vi "ADIS16470 Process AutoSPI DMA.vi"(8 "error in (no error)":T1, 9 "Bytes per Sample":numeric, 10 "Samples to Read":numeric) -> (0 "error out":T1, 1 "Timestamps":array[numeric], 2 "Data":array[numeric])   [LabVIEW 2019]
uses:
  <vilib>/Utility/error.llb/Error Cluster From Error Code.vi
  <vilib>/rvi/errors/niLvFpgaAdjustHostInterfaceError.vi
  <vilib>/rvi/interface/nirviMethod/nirviMethod.xnode
  <vilib>/Rock Robotics/SystemInterfaces/System/FPGA_SystemFRC FPGA Ref.ctl
  <vilib>/FPGAPlugInAG/Dynamic/niLvFpga_ReadFifo_Dynamic.vi
  <vilib>/rvi/errors/niLvFpgaMergeErrorWithErrorCode.vi
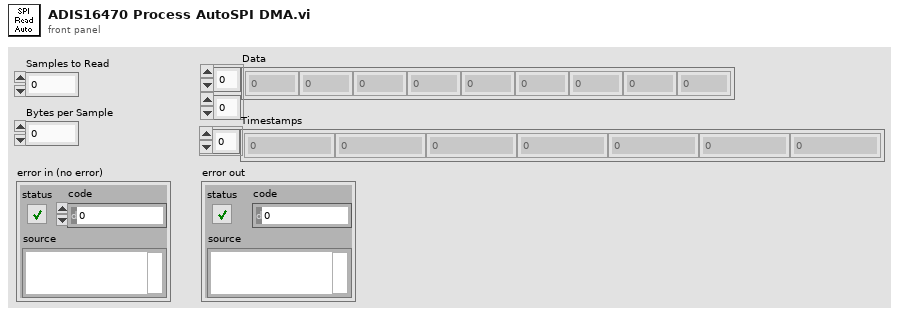
[diagram p1: front panel]
types:
  T1 = cluster{"source":string, "code":numeric, "status":boolean}
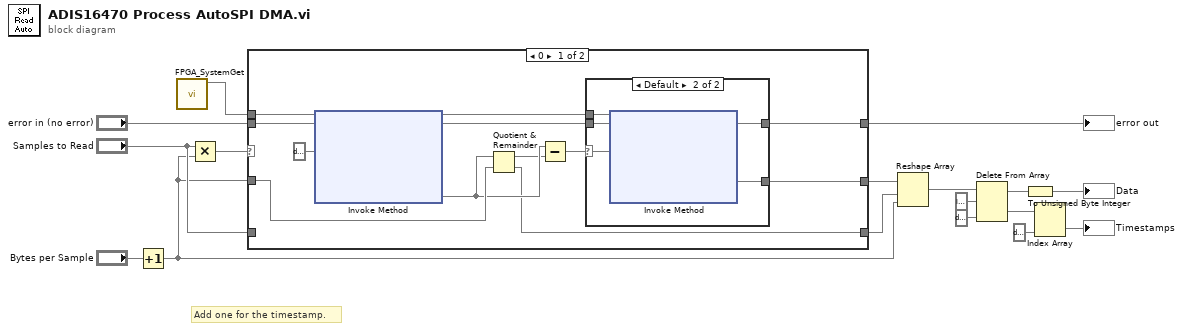
[diagram p0: block diagram]
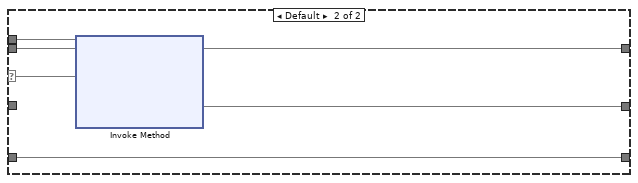
[diagram p3: hidden frame]
diagram:
  # "Add one for the timestamp."
  n1 = Increment(x="Bytes per Sample") -> (x+1=w9)
  n2 = call <vilib>:"FPGA_SystemGet.vi"() -> (3:w15)  [unwired: 11 in]
  n3 = Multiply(x="Samples to Read", y=w9) -> (x*y=w14)
  n4 = case shown="0" w14 {
    selector: w14 -> [_ w38]
    tunnel: [w24 w41] -> w17
    tunnel: "error in (no error)" -> [w29 w40]
    tunnel: w15 -> [w28 w39]
    tunnel: [w27 w37] -> w13
    tunnel: w9 -> [w23 _]
    tunnel: [w18 w36] -> w10
    tunnel: "Samples to Read" -> [_ w36]
    frame 0 {
      n5 = xnode "Invoke Method"(w28, w29, data[5B] ("Number of Elements")) -> (w26, w25, w22)  [unwired: 1 in, 1 out]
      n6 = Quotient & Remainder(x=w22, y=w23) -> (x-y*floor(x/y)=w21, floor(x/y)=w18)
      n7 = Subtract(x=w22, y=w21) -> (x-y=w20)
      n8 = case shown="Default" w20 {
        selector: w20 -> [_ w32]
        tunnel: [_ w31] -> w27
        tunnel: w26 -> [_ w35]
        tunnel: w25 -> [w30 w34]
        tunnel: [w30 w33] -> w24
        frame 0 {
        }
        frame Default {
          n9 = xnode "Invoke Method"(w35, w34, w32) -> (w33, w31)  [unwired: 1 in, 2 out]
        }
      }
    }
    frame Default {
      n10 = xnode "Invoke Method"(w39, w40, w38) -> (w41, w37)  [unwired: 1 in, 2 out]
    }
  }
  "error out" <- w17
  n11 = Reshape Array(w13, w10, w9) -> (w8)
  n12 = Delete From Array(array=w8, length=i32? 1, index (col)=data[5B] ("index (row)")) -> (deleted portion=w4, array with subset deleted=w6)  [unwired: 1 in]
  n13 = To Unsigned Byte Integer(number=w6) -> (unsigned 8bit integer=→"Data")
  n14 = Index Array(array=w4, index (col)=data[5B] ("index (row)")) -> (element=→"Timestamps")  [unwired: 1 in]
